vi "ReleaseCmdQueue.vi"(0 "cmdRef":T1, 11 "error in (no error)":errorcluster) -> (15 "error out":errorcluster)   [LabVIEW 2017, in "vsws.lvlib"]
uses:
  vsws.lvlib
  cmdRef.ctl
  cmd.ctl
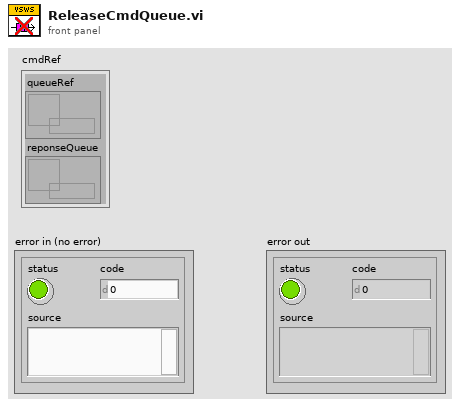
[diagram p1: front panel]
types:
  T1 = typedef "vsws.lvlib/cmdRef.ctl" = cluster{"queueRef":refnum<queue>, "reponseQueue":refnum<queue>}
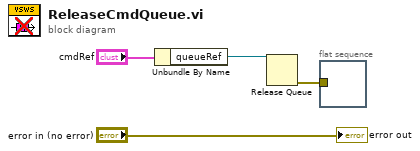
[diagram p0: block diagram]
diagram:
  n1 = Unbundle By Name("cmdRef") -> ("queueRef"=w3:refnum<queue>)
  n2 = Release Queue(queue=w3) -> (error out=w1:errorcluster)  [unwired: 2 in, 2 out]
  n3 = flat-sequence {
    tunnel: w1 -> [_]
    frame #0 {
    }
  }
  "error out" <- "error in (no error)"
